vi "Daq devices.vi"(7 "error in":errorcluster) -> (0 "error out":errorcluster, 1 "AO":string, 2 "AI array":string[](array[string]), 3 "DO":string, 5 "AI voltage":dbl[](array[numeric]))   [LabVIEW 2015]
uses:
  Daq Devices cmd.ctl
panel:
  in  "Daq Devices cmd":T1
  in  "Device":u16(ring) items=["ProCoDA", "Dev2"]
  in  "Max Voltage":T2(ring)
  in  "AI voltage":T3(array[ring])=[enum."0.5V", enum."0.5V", enum."0.5V", enum."0.5V"]
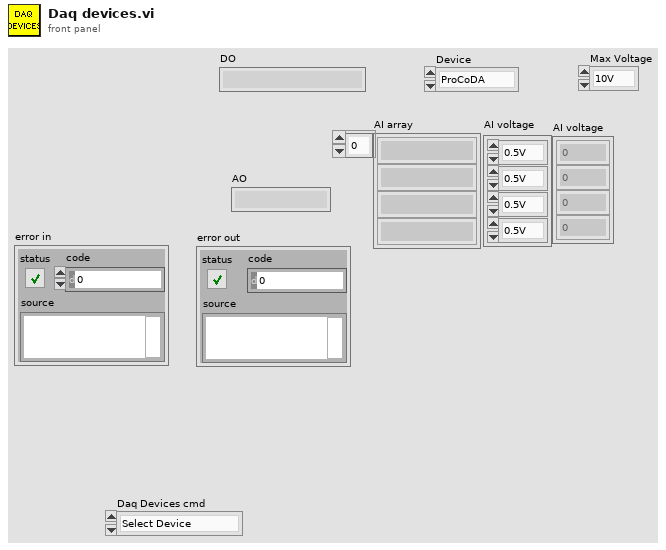
[diagram p1: front panel]
types:
  T1 = typedef "Daq Devices cmd.ctl" = enum16{"Select Device", "Read Channels"}
  T2 = enum16{"10V", "5V", "2.5V", "2V", "1.25V", "1V", "0.625V", "0.5V"}
  T3 = enum16{"10V", "5V", "2.5V", "2V", "1.25V", "1V", "0.625V", "0.5V"}[]
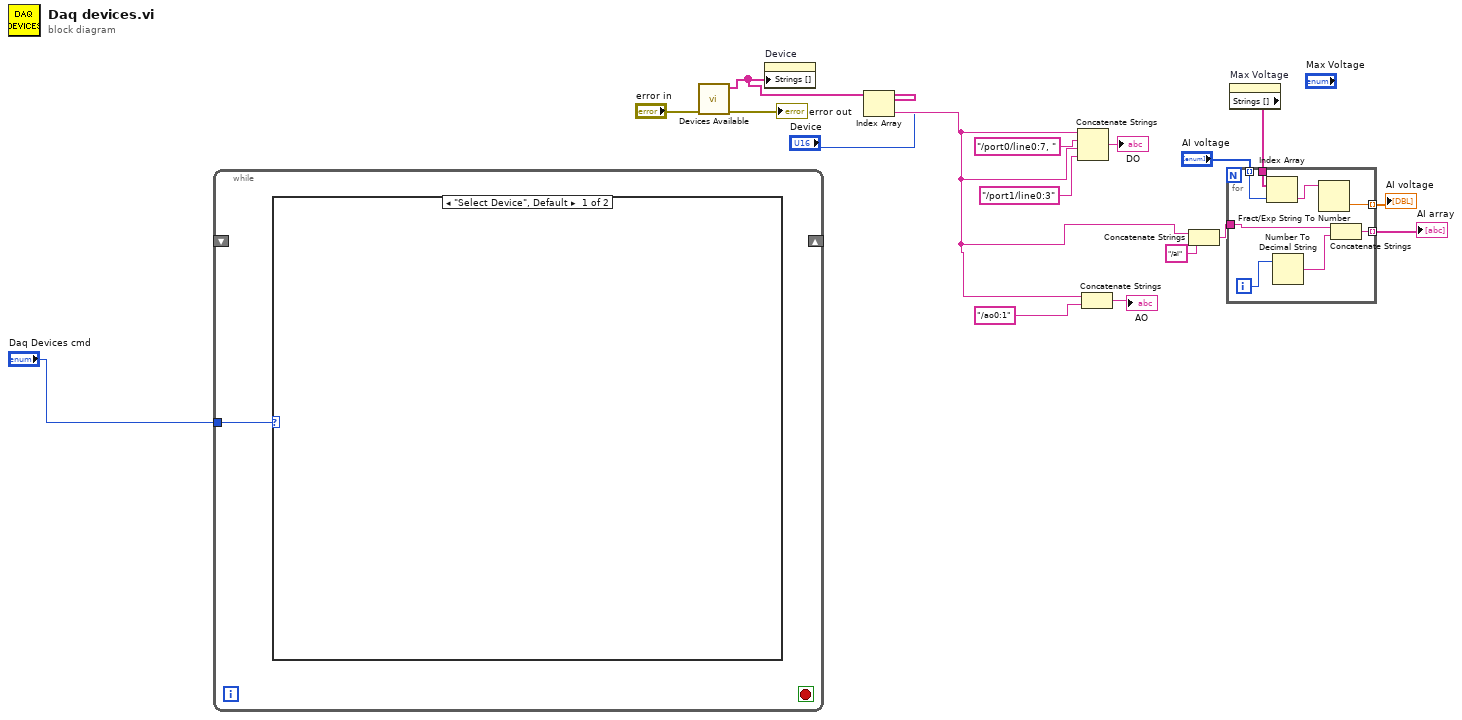
[diagram p0: block diagram]
diagram:
  n1 = while {
    shift-right: _ -> [_]
    shift-left: _ -> [_]
    tunnel: "Daq Devices cmd" -> [w18]
    stop <- _ stop-if-true
    n2 = case shown="\"Select Device\", Default" w18 {
      frame "Select Device", Default {
      }
      frame "Read Channels" {
      }
    }
  }
  n3 = call "Devices Available.vi"("error in (no error)"="error in") -> ("error out"=→"error out":errorcluster, "Devices"=w2:string[])  [unwired: 6 in, 3 out]
  n4 = property on="Device" class="Ring (strict)"("Strings []"=w2) -> ()  [unwired: 2 in, 2 out]
  n5 = Index Array(array=w2, index="Device") -> (element=w11:string)
  n6 = Concatenate Strings(w11, "/port0/line0:7, ", w11, "/port1/line0:3") -> (→"DO":string)
  n7 = Concatenate Strings(w11, "/ao0:1") -> (→"AO":string)
  n8 = Concatenate Strings(w11, "/ai") -> (w10:string)
  n9 = property on="Max Voltage" class="Enum (strict)"() -> ("Strings []"=w8:string[])  [unwired: 2 in, 2 out]
  n10 = for {
    tunnel: w10 -> [w26]
    tunnel: [w23] -> w9 mode=indexing
    tunnel: w8 -> [w22]
    tunnel: "AI voltage" -> [w21] mode=indexing
    tunnel: [w19] -> w6 mode=indexing
    i -> [w25]
    n11 = Index Array(array=w22, index=w21) -> (element=w20:string)
    n12 = Number To Decimal String(number=w25) -> (decimal integer string=w24:string)  [unwired: 1 in]
    n13 = Fract/Exp String To Number(string=w20) -> (number=w19:dbl)  [unwired: 3 in, 1 out]
    n14 = Concatenate Strings(w26, w24) -> (w23:string)
  }
  "AI array" <- w9
  "AI voltage" <- w6
